vi "Transition.vi"(8 "error in (no error)":errorcluster, 9 "Target State":refnum<class "State.lvclass">, 10 "Source State":refnum<class "State.lvclass">, 11 "Transition in":refnum<class "Transition.lvclass">) -> (0 "error out":errorcluster, 2 "State out":refnum<class "State.lvclass">, 3 "Transition out":refnum<class "Transition.lvclass">)   [LabVIEW 2024, in "Transition.lvlib" / "Transition.lvclass"]
uses:
  Transition.lvclass
  State/State/State.lvclass
  Transition.lvclass/Transition.ctl
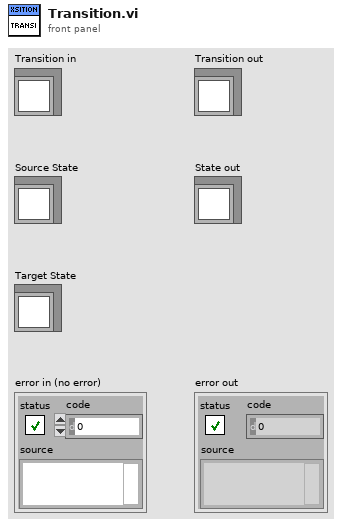
[diagram p1: front panel]
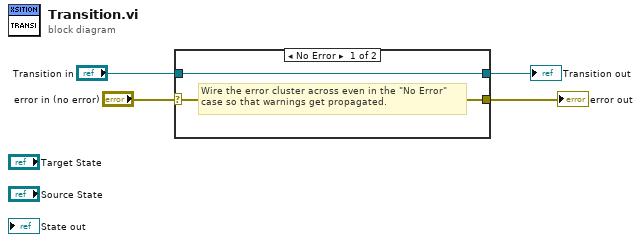
[diagram p0: block diagram]
diagram:
  n1 = case shown="No Error" "error in (no error)" {
    selector: "error in (no error)" -> [w5 w8]
    tunnel: [w5 w8] -> w3
    tunnel: [w6 w7] -> w1
    tunnel: "Transition in" -> [w6 w7]
    frame No Error {
      # "Wire the error cluster across even in the \"No Error\"\ncase so that warnings get propagated."
    }
    frame Error {
    }
  }
  "error out" <- w3
  "Transition out" <- w1
